vi "PDP Global.vi"() -> ()   [LabVIEW 2019]
panel:
  in  "FM Offset":dbl=0.5 format="%.1f"
  in  "FM Amplitude":dbl=0.5 format="%.1f"
  in  "Last Steps":i32
  in  "Last Mod":dbl format="%.2f"
  in  "Last Freq":dbl format="%.2f"
  out "x-Axis":dbl[](array[numeric]) format="%.3f"
  in  "Message Log":path=path "E:/log/pdp_messages.txt"
  in  "Setrate":dbl=0.5 format="%.2f"
  in  "Setpoint":dbl=77.085 format="%.3f"
  in  "Channel":i32
  in  "Cal Const":dbl=0.64413 format="%.2f"
  in  "ScanFreq":i32=100
  in  "ScanSteps":i32=500
  in  "RF Power":i32=280
  in  "RF Mod":i32=400
  in  "ScanSweeps":i32=100
  in  "Yale Gain":i32
  in  "RF Freq":dbl=213.0 format="%.2f"
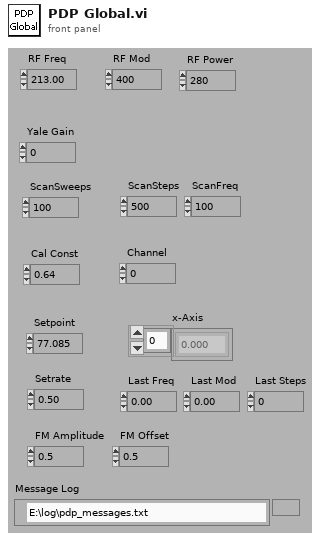
[diagram p1: front panel]
diagram:
